vi "Tektronix Model Check.vi"(8 "error in (no error)":errorcluster, 9 "Command String":string, 10 "Oscilloscope Model Tests (3: RF Model?)":u16(ring)=3 items=["Two-channel?", "Digital Model?", "Four-channel?", "RF Model?"], 11 "VISA resource name":refnum<visa-resource-name>) -> (0 "error out":errorcluster, 3 "VISA resource name out":refnum<visa-resource-name>)   [LabVIEW 2013, in "Tektronix DPO MSO 2000 4000 Series.lvlib"]
doc: "Performs a model check on the instrument to verify it supports the commandset that is being written to it. The VI also writes the input command to the instrument."
uses:
  Tektronix DPO MSO 2000 4000 Series.lvlib
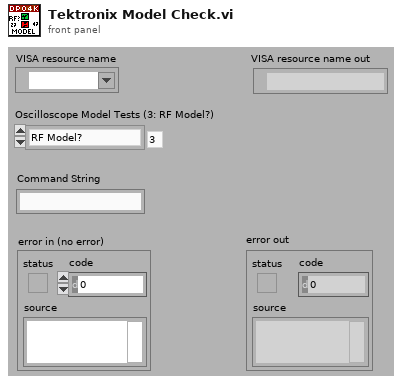
[diagram p1: front panel]
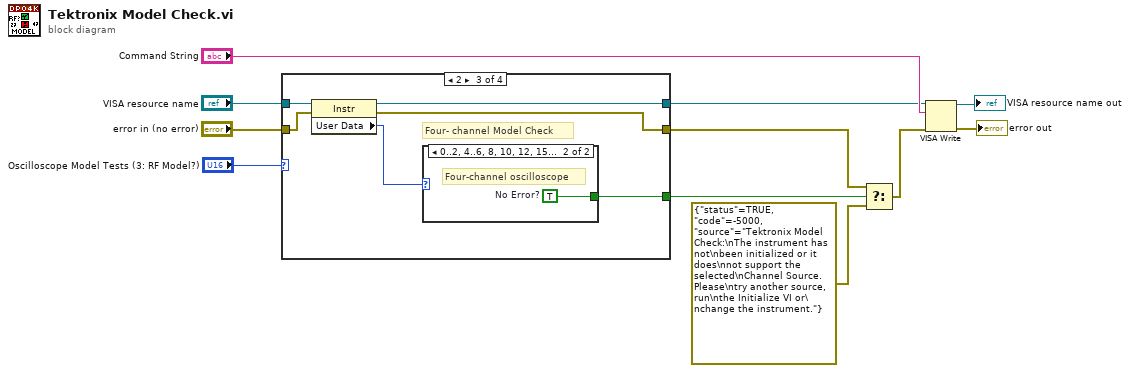
[diagram p0: block diagram]
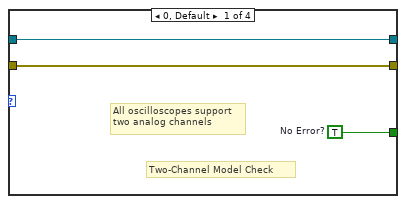
[diagram p2: hidden frame]
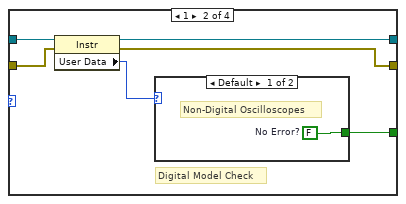
[diagram p3: hidden frame]
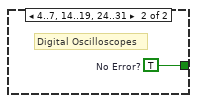
[diagram p4: hidden frame]
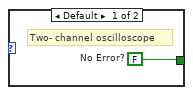
[diagram p5: hidden frame]
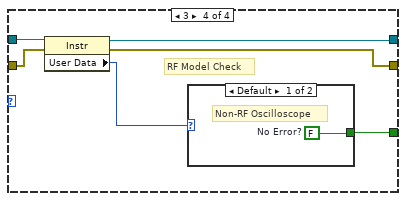
[diagram p6: hidden frame]
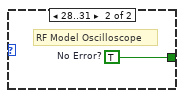
[diagram p7: hidden frame]
diagram:
  n1 = case shown="2" "Oscilloscope Model Tests (3: RF Model?)" {
    tunnel: "VISA resource name" -> [w14 w20 w28 w36]
    tunnel: "error in (no error)" -> [w13 w19 w27 w35]
    tunnel: [w14 w17 w26 w34] -> w5
    tunnel: [w13 w16 w25 w33] -> w4
    tunnel: [w12 w15 w23 w31] -> w3
    frame 0, Default {
      w12 = TRUE  # No Error?
      # "All oscilloscopes support\ntwo analog channels"
      # "Two-Channel Model Check"
    }
    frame 1 {
      # "Digital Model Check"
      n2 = property class="Instr"(reference=w20, error in=w19) -> (reference out=w17:refnum<visa-resource-name>, error out=w16:errorcluster, "User Data"=w18:u32)
      n3 = case shown="Default" w18 {
        tunnel: [w21 w22] -> w15
        frame Default {
          w21 = FALSE  # No Error?
          # "Non-Digital Oscilloscopes"
        }
        frame 4..7, 14..19, 24..31 {
          w22 = TRUE  # No Error?
          # "Digital Oscilloscopes"
        }
      }
    }
    frame 2 {
      # "Four- channel Model Check"
      n4 = property class="Instr"(reference=w28, error in=w27) -> (reference out=w26:refnum<visa-resource-name>, error out=w25:errorcluster, "User Data"=w24:u32)
      n5 = case shown="0..2, 4..6, 8, 10, 12, 15, 17, 19..21, 23..25, 28..31" w24 {
        tunnel: [w29 w30] -> w23
        frame Default {
          w29 = FALSE  # No Error?
          # "Two- channel oscilloscope"
        }
        frame 0..2, 4..6, 8, 10, 12, 15, 17, 19..21, 23..25, 28..31 {
          w30 = TRUE  # No Error?
          # "Four-channel oscilloscope"
        }
      }
    }
    frame 3 {
      # "RF Model Check"
      n6 = property class="Instr"(reference=w36, error in=w35) -> (reference out=w34:refnum<visa-resource-name>, error out=w33:errorcluster, "User Data"=w32:u32)
      n7 = case shown="Default" w32 {
        tunnel: [w37 w38] -> w31
        frame Default {
          w37 = FALSE  # No Error?
          # "Non-RF Oscilloscope"
        }
        frame 28..31 {
          w38 = TRUE  # No Error?
          # "RF Model Oscilloscope"
        }
      }
    }
  }
  n8 = Select(t=w4, s=w3, f=errorcluster {"status"=TRUE, "code"=-5000, "source"="Tektronix Model Check:\nThe instrument has not\nbeen initialized or it does\nnot support the selected\nChannel Source. Please\ntry another source, run\nthe Initialize VI or\nchange the instrument."} ("error out")) -> (s? t:f=w9:errorcluster)
  n9 = VISA Write(VISA resource name=w5, write buffer="Command String", error in (no error)=w9) -> (VISA resource name out=→"VISA resource name out":refnum<visa-resource-name>, error out=→"error out":errorcluster)  [unwired: 1 out]
